vi "Position.vi"(8 "error in (no error)":errorcluster, 10 "Panel VI":refnum<vi>, 11 "Persistent Position in":refnum<class "Persistent Position.lvclass">) -> (0 "error out":errorcluster, 2 "Open Maximized?":bool)   [LabVIEW 2017, in "MGI-Panel Manager.lvlib" / "Persistent Position.lvclass"]
doc: "Positions the window. By default the Panel VI will be centered.\n\n----\nPlease see the following web address for additional documentation and tutorial information:\nhttp://www.mooregoodideas.com/mgi-panel-manager/\n\nAuthor: Derek Trepanier\n\nCopyright (c) 2018, Moore Good Ideas, Inc.\n\nAll rights reserved.\n\nRedistribution and use in source and binary forms, with or without modification, are permitted provided that the following conditions are met:\n\n * Redistributions of source code must retain the above copyright notice, this list of conditions and the following disclaimer.\n * Redistributions in binary form must reproduce the above copyright notice, this list of conditions and the following disclaimer in the documentation and/or other materials provided with the distribution.\n * Neither the name of Moore Good Ideas, Inc. nor the names of its contributors may be used to endorse or promote products derived from this software without specific prior written permission.\n\nTHIS SOFTWARE IS PROVIDED BY THE COPYRIGHT HOLDERS AND CONTRIBUTORS \"AS IS\" AND ANY EXPRESS OR IMPLIED WARRANTIES, INCLUDING, BUT NOT LIMITED TO, THE IMPLIED WARRANTIES OF MERCHANTABILITY AND FITNESS FOR A PARTICULAR PURPOSE ARE DISCLAIMED. IN NO EVENT SHALL THE COPYRIGHT OWNER OR CONTRIBUTORS BE LIABLE FOR ANY DIRECT, INDIRECT, INCIDENTAL, SPECIAL, EXEMPLARY, OR CONSEQUENTIAL DAMAGES (INCLUDING, BUT NOT LIMITED TO, PROCUREMENT OF SUBSTITUTE GOODS OR SERVICES; LOSS OF USE, DATA, OR PROFITS; OR BUSINESS INTERRUPTION) HOWEVER CAUSED AND ON ANY THEORY OF LIABILITY, WHETHER IN CONTRACT, STRICT LIABILITY, OR TORT (INCLUDING NEGLIGENCE OR OTHERWISE) ARISING IN ANY WAY OUT OF THE USE OF THIS SOFTWARE, EVEN IF ADVISED OF THE POSSIBILITY OF SUCH DAMAGE."
uses:
  Persistent Position.lvclass
  Persistent Position.lvclass/Persistent Position.ctl
  <vilib>/Utility/config.llb/Read Key (String).vi
  Window Position.lvclass
  <vilib>/Utility/config.llb/NI_LVConfig.lvlib
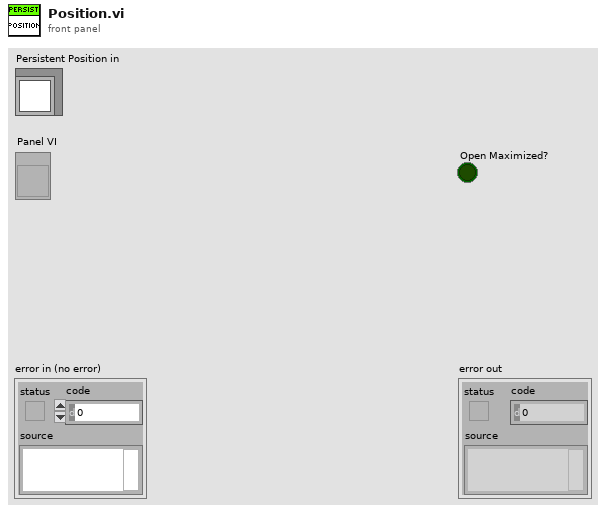
[diagram p1: front panel]
types:
  T1 = typedef "NI_LVConfig.lvlib/Config Data RefNum.ctl" = refnum<k1>
  T2 = cluster{"[0]":i16, "[1]":i16, "[2]":i16, "[3]":i16}
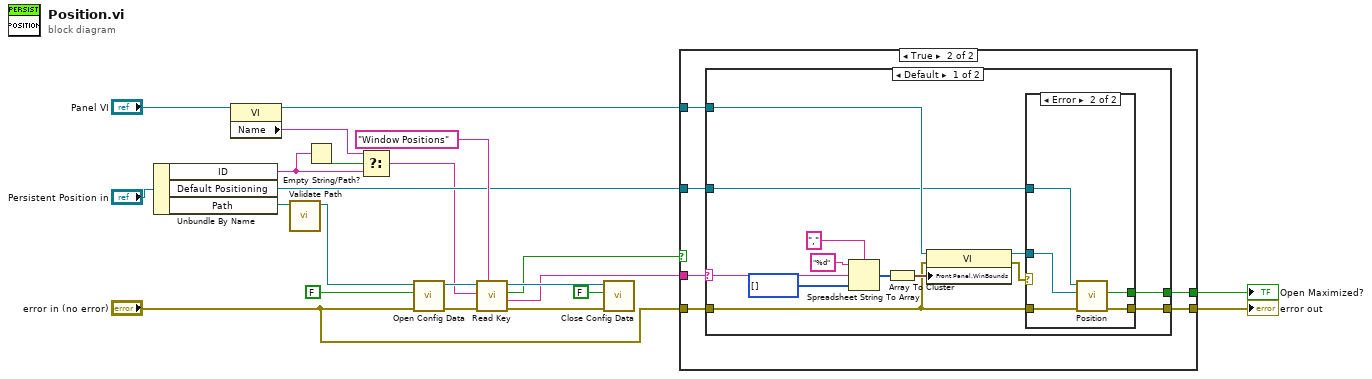
[diagram p0: block diagram]
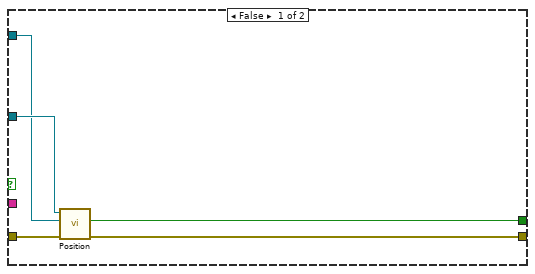
[diagram p2: hidden frame]
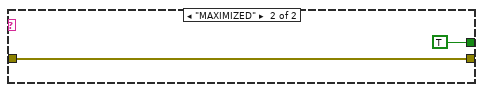
[diagram p4: hidden frame]
diagram:
  n1 = Unbundle By Name("Persistent Position in") -> ("ID"=w3:string, "Default Positioning"=w9:refnum<class "Window Position.lvclass">, "Path"=w21:path)
  n2 = property class="VI"(reference="Panel VI") -> (reference out=w7:refnum<vi>, "Name"=w2:string)  [unwired: 1 in, 1 out]
  n3 = call "Validate Path.vi"("Path in"=w21) -> ("Path out"=w20:path)  [unwired: 10 in]
  n4 = Empty String/Path?(string/path=w3) -> (empty?=w4:bool)
  n5 = Select(t=w2, s=w4, f=w3) -> (s? t:f=w1:string)
  n6 = call <vilib>:"Open Config Data.vi"("error in (no error)"="error in (no error)", "create file if necessary (T)"=FALSE, "configuration file path"=w20) -> ("error out"=w19:errorcluster, "refnum"=w17:T1)  [unwired: 6 in, 1 out]
  n7 = call-poly <vilib>:"Read Key.vi"("section"="Window Positions", "error in (no error)"=w19, "key"=w1, "refnum"=w17) -> ("error out"=w15:errorcluster, "value"=w6:string, "found?"=w11:bool, "refnum out"=w16:T1)  [unwired: 4 in]
  n8 = call <vilib>:"Close Config Data.vi"("error in (no error)"=w15, "write file if changed (T)"=FALSE, "refnum"=w16) -> ()  [unwired: 7 in, 2 out]
  n9 = case shown="True" w11 {
    tunnel: [w26 w30] -> w10
    tunnel: "error in (no error)" -> [w27 w29]
    tunnel: w9 -> [w25 w28]
    tunnel: [w24 w31] -> w8
    tunnel: w7 -> [w23 w32]
    tunnel: w6 -> [_ w33]
    frame False {
      n10 = call-dynamic "Position.vi"("error in (no error)"=w27, "Panel VI"=w23, "Window Position in"=w25) -> ("error out"=w26:errorcluster, "Open Maximized?"=w24:bool)  [unwired: 7 in]
    }
    frame True {
      n11 = case shown="Default" w33 {
        selector: w33 -> [w45 _]
        tunnel: w32 -> [w46 _]
        tunnel: [w35 TRUE] -> w31
        tunnel: [w36 w53] -> w30
        tunnel: w29 -> [w37 w53]
        tunnel: w28 -> [w34 _]
        frame Default {
          n12 = Spreadsheet String To Array(delimiter (Tab)=",", format string="%d", spreadsheet string=w45, array type (2D Dbl)=i16[] []) -> (array=w42:i16[])
          n13 = Array To Cluster(array=w42) -> (cluster=w41:T2)
          n14 = property class="VI"(reference=w46, error in=w37, "Front Panel.WinBounds"=w41) -> (reference out=w39:refnum<vi>, error out=w38:errorcluster)
          n15 = case shown="Error" w38 {
            tunnel: w39 -> [_ w49]
            tunnel: w37 -> [w47 w52]
            tunnel: [w47 w51] -> w36
            tunnel: [_ w50] -> w35
            tunnel: w34 -> [_ w48]
            frame No Error {
            }
            frame Error {
              n16 = call-dynamic "Position.vi"("error in (no error)"=w52, "Panel VI"=w49, "Window Position in"=w48) -> ("error out"=w51:errorcluster, "Open Maximized?"=w50:bool)  [unwired: 7 in]
            }
          }
        }
        frame "MAXIMIZED" {
        }
      }
    }
  }
  "error out" <- w10
  "Open Maximized?" <- w8
